vi "uTTA_Main_Temperature_Control.vi"() -> ()   [LabVIEW 2021]
uses:
  uTTA_Device_Driver/uTTA_Controls/CTL_uTTA_MeasurementStates.ctl
  <vilib>/Utility/miscctls.llb/LVPointTypeDef.ctl
  uTTA_Device_Driver/uTTA_Controls/CTL_uTTA_OperatingMode.ctl
  uTTA_Device_Driver/uTTA_Controls/CTL_uTTA_AnalogParameter.ctl
  <vilib>/Utility/error.llb/DialogType.ctl
  uTTA_Device_Driver/uTTA_SubVi/Serial_Port/uTTA_GV_Serial_Monitor.vi
panel:
  out "Updated":dbl
  out "Stable Time":dbl
  in  "Set Point":dbl
  out "Temperature":dbl
  in  "Update_Time":dbl=0.5
  out "uTTA_CalData":T1(array[cluster])
  out "ADC Overrange":bool[](array[boolean])
  out "GUI State":string="EXIT"
  out "Heating Power":dbl format="%#_3pW"
  out "Total Runtime":timestamp=timestamp(-3599.4283056259155 s since 1904-01-01) format="%<%H:%M:%S>T"
  out "Measurement Started":timestamp=timestamp(3793474800.1504135 s since 1904-01-01) format="%<%X>T"
  out "Diode Voltages":T2(graph)
  out "Temp":T3(graph)
  out "Measurement State":T4=enum."Cooling" caption="uTTA State"
  in  "Tab Control":T5(tab)
  out "ADC1L_Range":dbl caption="Lower Limit" format="%.2pV"
  out "ADC1H_Range":dbl caption="Upper Limit" format="%.2pV"
  in  "CH1-2 Offset":dbl(slide)=-0.4 scale=-2.5..2.5 scale format="%.2pV"
  out "ADC0H_Range":dbl caption="Upper Limit" format="%.2pV"
  out "ADC0L_Range":dbl caption="Lower Limit" format="%.2pV"
  in  "CH0 Offset":dbl(slide)=-0.63 scale=-2.5..2.5 scale format="%.2pV"
  in  "Sense Current":dbl(slide)=0.01 caption="CH0" min=0.0 max=0.011 step=0.0001 scale=0.0..0.011 scale format="%.1pA"
  in  "µTTA Port":refnum<visa-resource-name>="COM3"
  in  "Connect":bool
  in  "Disconnect":bool
  in  "Heating":u16(ring) items=["PGA = 0", "PGA = 1", "PGA = 2", "PGA = 3"]
  in  "Start":bool
  in  "Stop":bool
  in  "Autoscroll":bool
  out "Serial Monitor OUT":string
  in  "Serial Monitor":bool
  out "RunTime Error":errorcluster
  out "Exit Error":errorcluster
  out "Device Info":string
  # "Measurement\nRange"
  # "Measurement \nRange"
  # "Channel Offset"
  # "Sense Current"
  # "PGA"
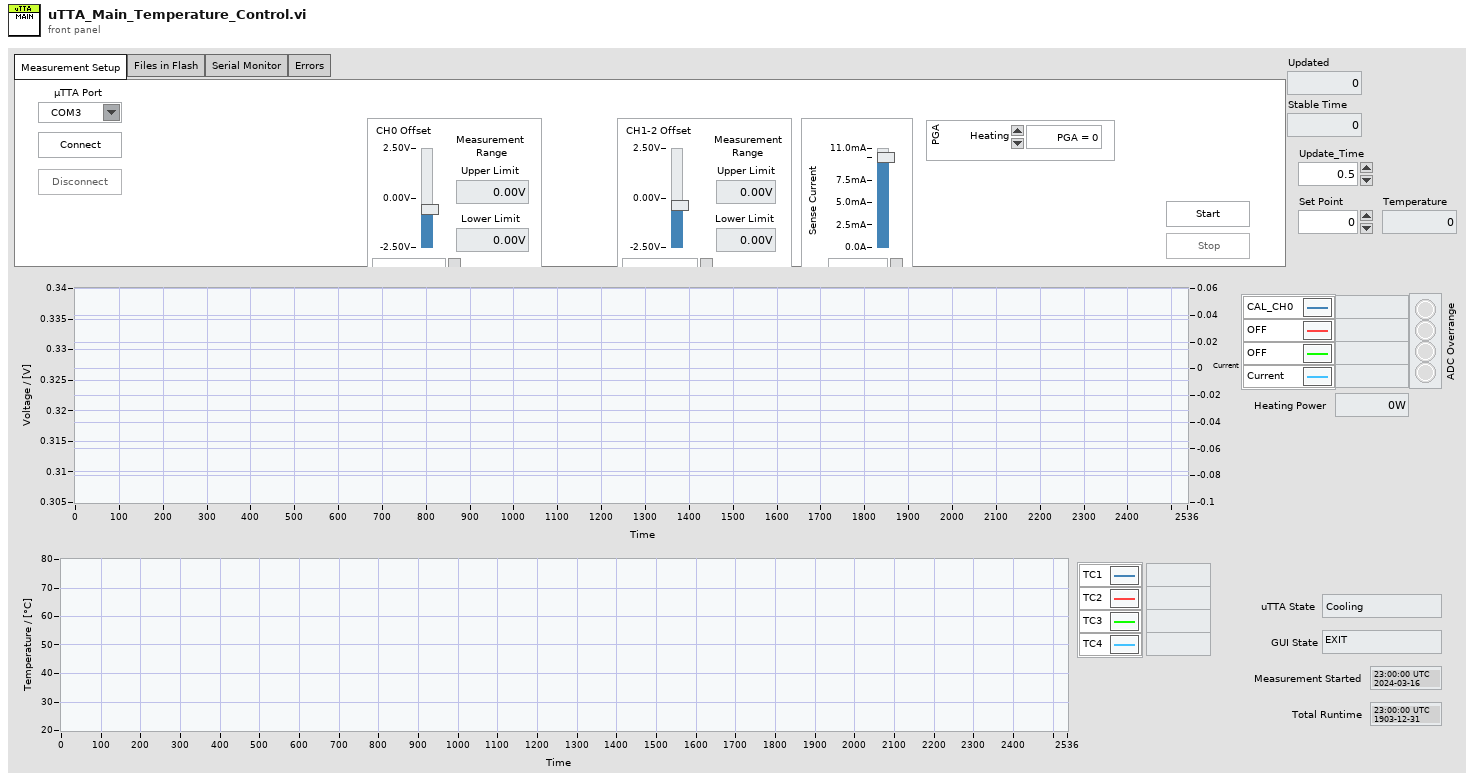
[diagram p1: front panel]
types:
  T1 = cluster{"Diff Gain":dbl, "Offset":dbl[], "Gain":dbl[]}[]
  T2 = cluster{"Diode Voltage":dbl, "Diode Voltage":dbl, "Diode Voltage":dbl, "Current":dbl}
  T3 = cluster{"Diode Voltage":dbl, "Diode Voltage":dbl, "Diode Voltage":dbl, "Diode Voltage":dbl}
  T4 = typedef "CTL_uTTA_MeasurementStates.ctl" = enum16{"Idle", "Init", "GPPowerCheck", "InitMeasFile", "Preheating", "PrepHeating", "Heating", "PrepCooling", "Cooling", "Deinit", "CloseLog", "Cal_Init", "Cal_GDPowerOn", "Cal_GDPowerCheck", "Cal_Cal", "Cal_Deinit"}
  T5 = enum32{"Measurement Setup", "Files in Flash", "Serial Monitor", "Errors"}
  T6 = typedef "LVPointTypeDef.ctl" = cluster{"Horizontal":i16, "Vertical":i16}
  T7 = typedef "CTL_uTTA_AnalogParameter.ctl" = enum16{"ISEN", "SPARE", "VOFF"}
  T8 = enum8{"Enabled", "Disabled", "Disabled and Grayed Out"}
  T9 = typedef "CTL_uTTA_OperatingMode.ctl" = enum16{"NORMAL", "TEST_MODE", "TEMP_CONTROL"}
  T10 = cluster{"Diode Voltage":dbl, "Diode Voltage":dbl, "Diode Voltage":dbl, "Current":dbl}[]
  T11 = cluster{"Diode Voltage":dbl, "Diode Voltage":dbl, "Diode Voltage":dbl, "Diode Voltage":dbl}[]
  T12 = cluster{"Measurement State":T4, "Diode Voltages":dbl[], "Current":dbl, "Temperatures":dbl[], "NewData":bool, "ADC Overrange":bool[]}
  T13 = typedef "DialogType.ctl" = u16
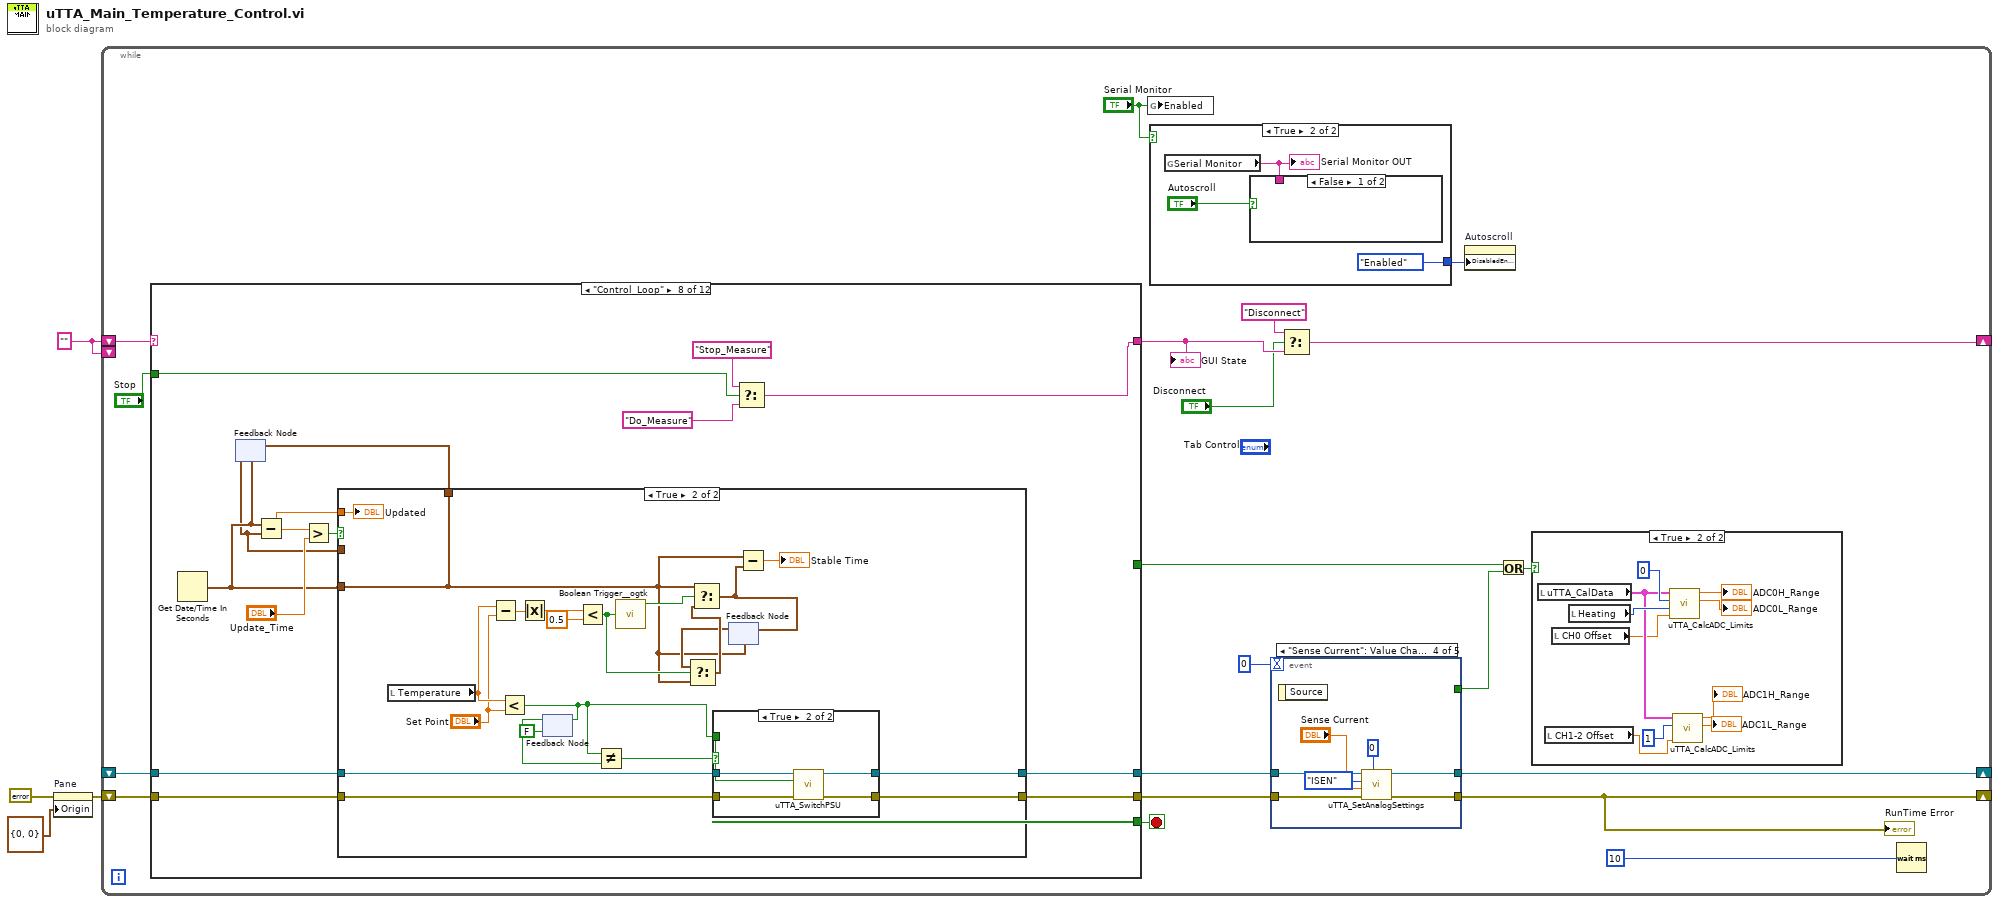
[diagram p0: block diagram]
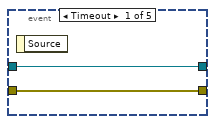
[diagram p3: hidden frame]
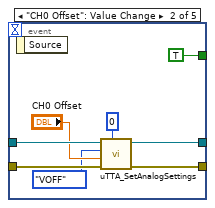
[diagram p4: hidden frame]
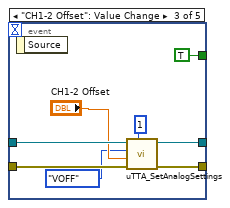
[diagram p5: hidden frame]
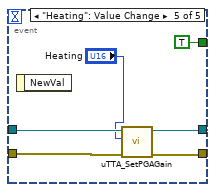
[diagram p6: hidden frame]
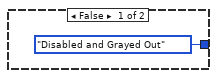
[diagram p7: hidden frame]
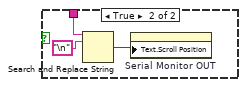
[diagram p8: hidden frame]
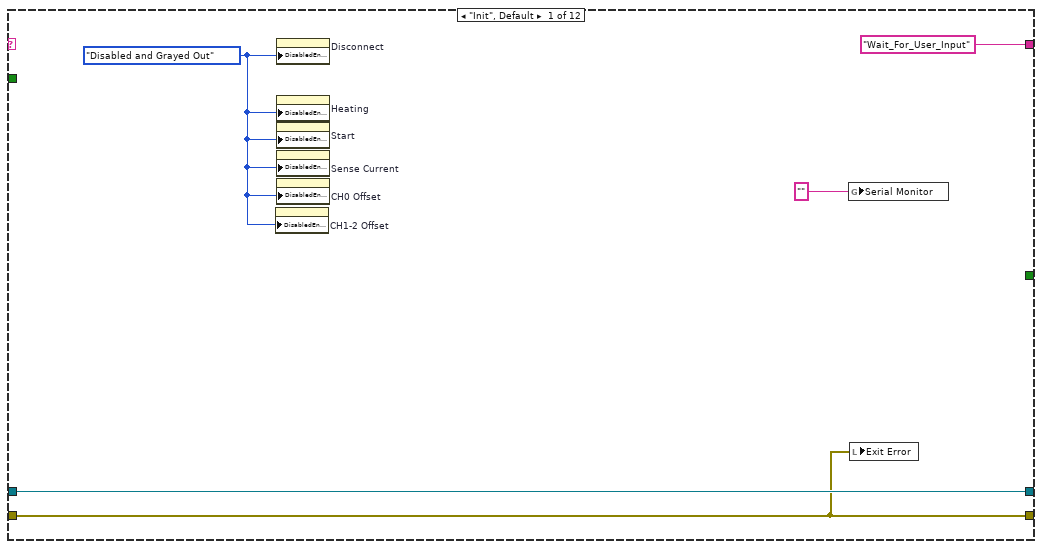
[diagram p9: hidden frame]
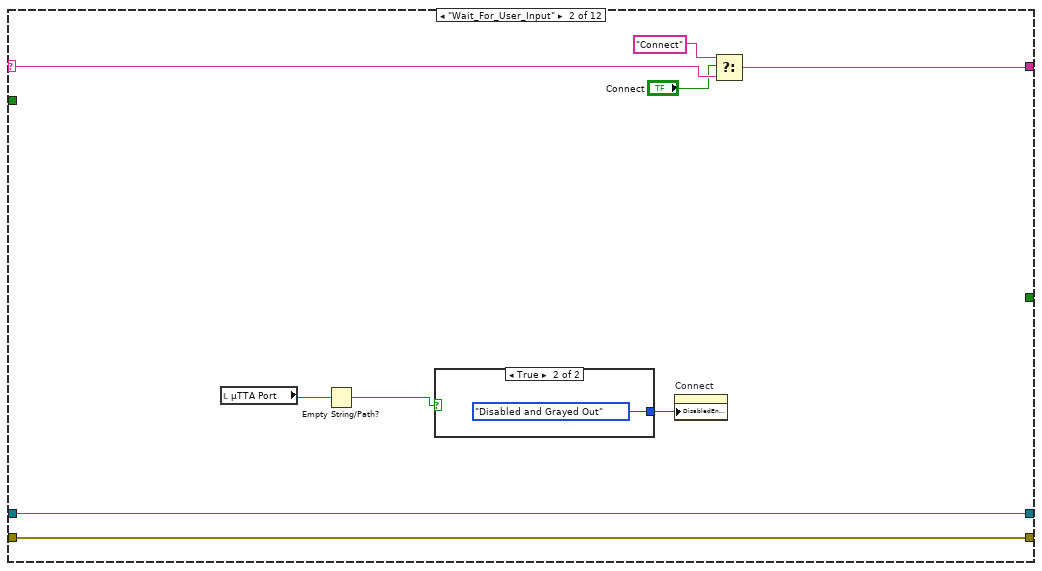
[diagram p10: hidden frame]
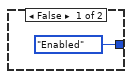
[diagram p11: hidden frame]
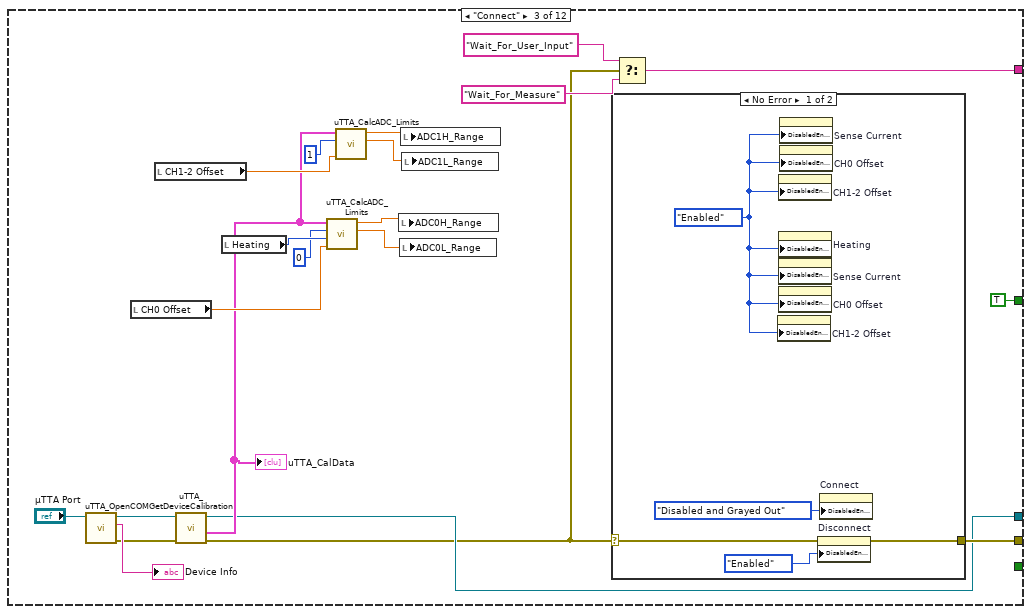
[diagram p12: hidden frame]
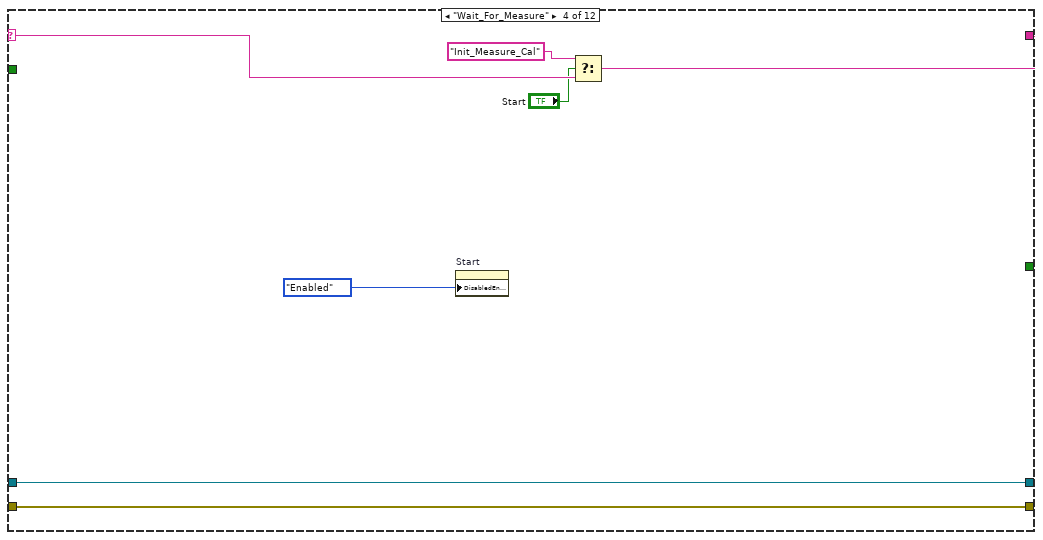
[diagram p14: hidden frame]
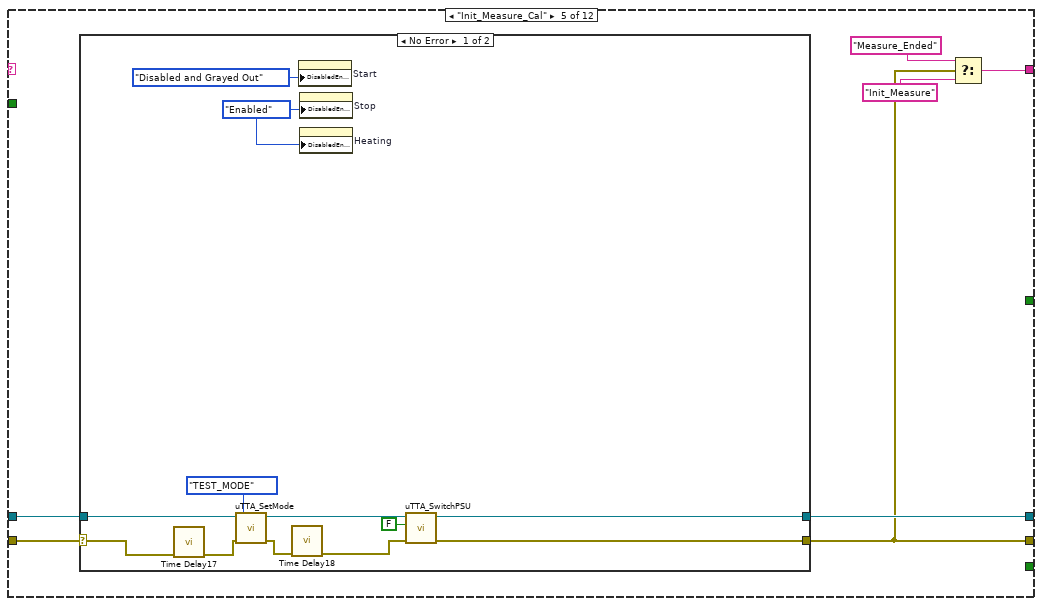
[diagram p15: hidden frame]
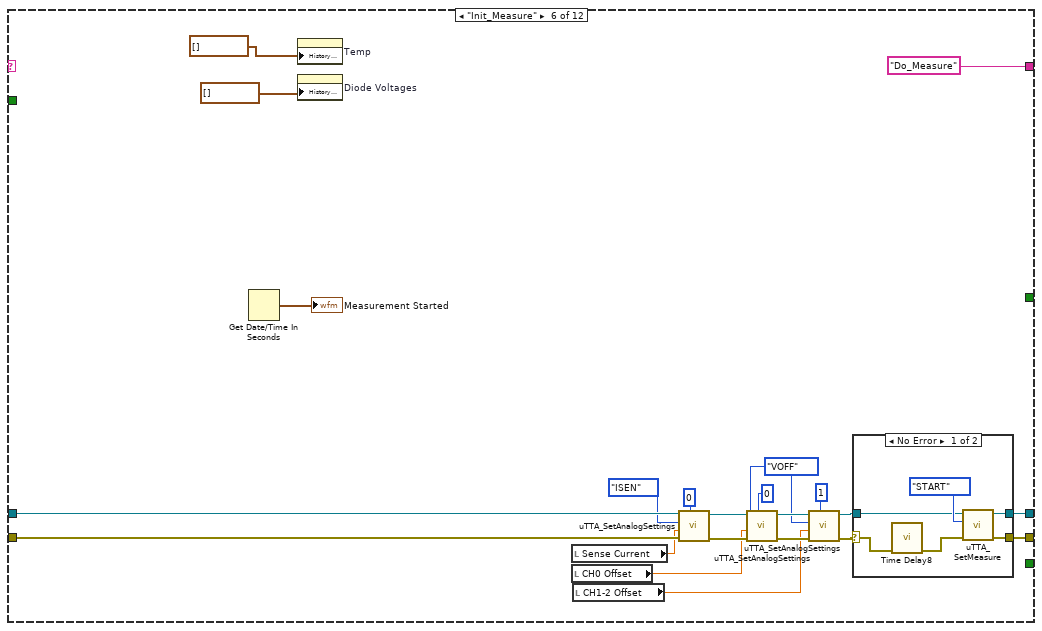
[diagram p17: hidden frame]
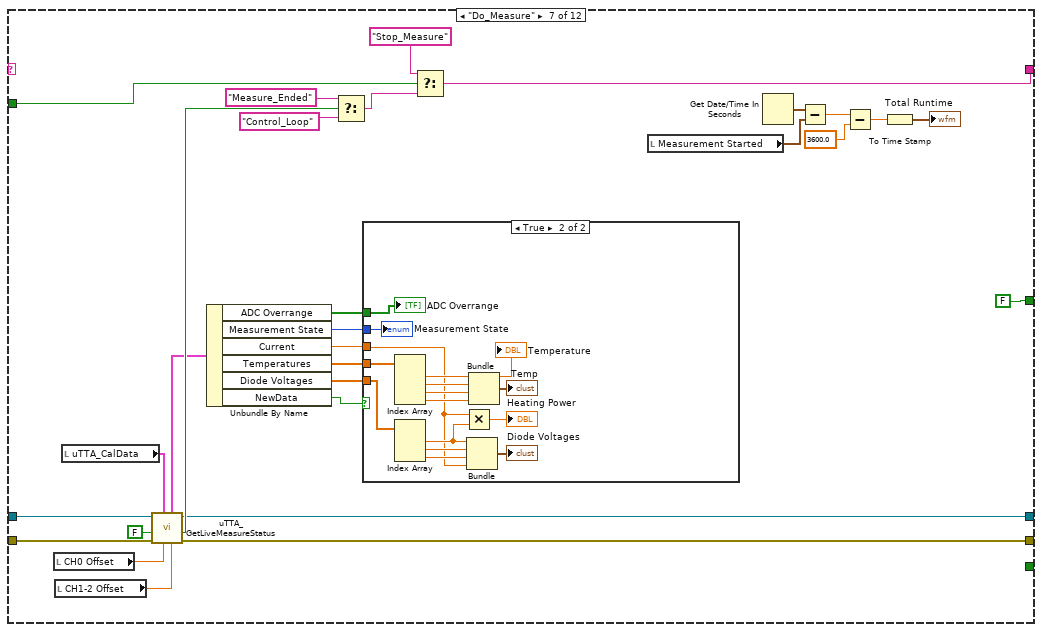
[diagram p19: hidden frame]
diagram:
  w1 = "" ("Identity")
  n1 = property on="Pane" class="Pane"(error in=errorcluster {"status"=FALSE, "code"=0, "source"=""} ("error out"), "Origin"=T6 {"Horizontal"=0, "Vertical"=0}) -> (error out=w2:errorcluster)  [unwired: 1 in, 1 out]
  n2 = while {
    shift-right: [w18] -> _
    shift-left: w1 -> [w24]
    shift-right: [w10] -> _
    shift-left: _ -> [w23]
    shift-right: [w8] -> _
    shift-left: w2 -> [w22]
    shift-left: w1 -> [_]
    stop <- w21 stop-if-true
    n3 = case shown="\"Control_Loop\"" w24 {
      selector: w24 -> [_ w85 _ w121 _ _ _ _ _ _ _ w287]
      tunnel: ["Wait_For_User_Input" w86 w104 w120 w124 "Do_Measure" ("t") w190 w223 "Measure_Ended" ("t") "Wait_For_Measure" ("t") "EXIT" w287] -> w19
      tunnel: [w76 w83 w90 w118 w129 w165 w181 w228 w265 w272 refnum<visa-resource-name> refnum ("VISA out") w286] -> w11
      tunnel: w23 -> [w76 w83 _ w118 w128 w160 w202 w229 w267 w272 w281 w286]
      tunnel: w22 -> [w75 w82 _ w116 w127 w161 w201 w226 w266 w271 w282 w285]
      tunnel: [w75 w82 w107 w116 w123 w164 w180 w227 w264 w271 w278 w285] -> w9
      tunnel: [_ _ _ _ _ _ _ _ _ _ _ TRUE] -> w21
      tunnel: "Stop" -> [_ _ _ _ _ _ w193 w224 _ _ _ _]
      tunnel: [_ _ TRUE _ _ _ FALSE _ _ _ _ _] -> w5
      frame "Init", Default {
        w73 = T8."Disabled and Grayed Out" ("Disabled")
        n4 = property on="CH1-2 Offset" class="Slide (strict)"("DisabledEnum"=w73) -> ()  [unwired: 2 in, 2 out]
        n5 = property on="Disconnect" class="Bool"("DisabledEnum"=w73) -> ()  [unwired: 2 in, 2 out]
        n6 = property on="Heating" class="Ring (strict)"("DisabledEnum"=w73) -> ()  [unwired: 2 in, 2 out]
        n7 = property on="Start" class="Bool"("DisabledEnum"=w73) -> ()  [unwired: 2 in, 2 out]
        n8 = property on="Sense Current" class="Slide (strict)"("DisabledEnum"=w73) -> ()  [unwired: 2 in, 2 out]
        n9 = property on="CH0 Offset" class="Slide (strict)"("DisabledEnum"=w73) -> ()  [unwired: 2 in, 2 out]
        n10 = global write "uTTA_GV_Serial_Monitor.vi" "Serial Monitor"("" ("Received")) -> ()
        n11 = local write "Exit Error"(w75) -> ()
      }
      frame "Wait_For_User_Input" {
        n12 = local read "µTTA Port"() -> (w81:refnum<visa-resource-name>)
        n13 = Empty String/Path?(string/path=w81) -> (empty?=w78:bool)
        n14 = case shown="True" w78 {
          tunnel: [T8."Enabled" ("Disabled") T8."Disabled and Grayed Out" ("Disabled")] -> w79
          frame False {
          }
          frame True {
          }
        }
        n15 = property on="Connect" class="Bool"("DisabledEnum"=w79) -> ()  [unwired: 2 in, 2 out]
        n16 = Select(t="Connect", s="Connect", f=w85) -> (s? t:f=w86:string)
      }
      frame "Connect" {
        n17 = call "uTTA_OpenCOM.vi"("VISA in"="µTTA Port") -> ("error out"=w93:errorcluster, "Identity"=→"Device Info":string, "VISA out"=w94:refnum<visa-resource-name>)  [unwired: 8 in]
        n18 = local read "CH0 Offset"() -> (w96:dbl)
        n19 = local read "CH1-2 Offset"() -> (w101:dbl)
        n20 = call "uTTA_GetDeviceCalibration.vi"("error in"=w93, "VISA Refnum in"=w94) -> ("error out"=w89:errorcluster, "uTTA_CalData"=w92:T1, "VISA Refnum out"=w90:refnum<visa-resource-name>)  [unwired: 2 in, 1 out]
        "uTTA_CalData" <- w92
        n21 = local read "Heating"() -> (w103:u16)
        n22 = call "uTTA_CalcADC_Limits.vi"("Offset Voltage"=w96, "PGA_Setting"=w103, "Channel Number"=u32 0, "uTTA_CalData"=w92) -> ("Range Low End"=w97:dbl, "Range High End"=w98:dbl)  [unwired: 6 in]
        n23 = call "uTTA_CalcADC_Limits.vi"("Offset Voltage"=w101, "Channel Number"=u32 1, "uTTA_CalData"=w92) -> ("Range Low End"=w99:dbl, "Range High End"=w100:dbl)  [unwired: 7 in]
        n24 = local write "ADC0H_Range"(w98) -> ()
        n25 = local write "ADC0L_Range"(w97) -> ()
        n26 = local write "ADC1H_Range"(w100) -> ()
        n27 = local write "ADC1L_Range"(w99) -> ()
        n28 = case shown="No Error" w89 {
          selector: w89 -> [w112 w115]
          tunnel: [w113 w115] -> w107
          frame No Error {
            w110 = T8."Enabled" ("Disabled")
            n29 = property on="CH1-2 Offset" class="Slide (strict)"("DisabledEnum"=w110) -> ()  [unwired: 2 in, 2 out]
            n30 = property on="CH1-2 Offset" class="Slide (strict)"("DisabledEnum"=w110) -> ()  [unwired: 2 in, 2 out]
            n31 = property on="Heating" class="Ring (strict)"("DisabledEnum"=w110) -> ()  [unwired: 2 in, 2 out]
            n32 = property on="Sense Current" class="Slide (strict)"("DisabledEnum"=w110) -> ()  [unwired: 2 in, 2 out]
            n33 = property on="CH0 Offset" class="Slide (strict)"("DisabledEnum"=w110) -> ()  [unwired: 2 in, 2 out]
            n34 = property on="Sense Current" class="Slide (strict)"("DisabledEnum"=w110) -> ()  [unwired: 2 in, 2 out]
            n35 = property on="CH0 Offset" class="Slide (strict)"("DisabledEnum"=w110) -> ()  [unwired: 2 in, 2 out]
            n36 = property on="Disconnect" class="Bool"(error in=w112, "DisabledEnum"=T8."Enabled" ("Disabled")) -> (error out=w113:errorcluster)  [unwired: 1 in, 1 out]
            n37 = property on="Connect" class="Bool"("DisabledEnum"=T8."Disabled and Grayed Out" ("Disabled")) -> ()  [unwired: 2 in, 2 out]
          }
          frame Error {
          }
        }
        n38 = Select(t="Wait_For_User_Input", s=w89, f="Wait_For_Measure" ("t")) -> (s? t:f=w104:string)
      }
      frame "Wait_For_Measure" {
        n39 = property on="Start" class="Bool"("DisabledEnum"=T8."Enabled" ("Disabled")) -> ()  [unwired: 2 in, 2 out]
        n40 = Select(t="Init_Measure_Cal", s="Start", f=w121) -> (s? t:f=w120:string)
      }
      frame "Init_Measure_Cal" {
        n41 = case shown="No Error" w127 {
          selector: w127 -> [w138 w142]
          tunnel: w128 -> [w137 w143]
          tunnel: [w132 w143] -> w129
          tunnel: [w131 w142] -> w123
          frame No Error {
            w136 = T8."Enabled" ("Disabled")
            n42 = call "Time Delay17"("error in (no error)"=w138) -> ("error out"=w139:errorcluster)  [unwired: 10 in]
            n43 = call "uTTA_SetMode.vi"("error in"=w139, "OperatingMode"=CTL_uTTA_OperatingMode."TEST_MODE", "VISA Refnum in"=w137) -> ("error out"=w140:errorcluster, "VISA Refnum out"=w134:refnum<visa-resource-name>)  [unwired: 2 in, 1 out]
            n44 = call "Time Delay18"("error in (no error)"=w140) -> ("error out"=w133:errorcluster)  [unwired: 10 in]
            n45 = property on="Start" class="Bool"("DisabledEnum"=T8."Disabled and Grayed Out" ("Disabled")) -> ()  [unwired: 2 in, 2 out]
            n46 = property on="Stop" class="Bool"("DisabledEnum"=w136) -> ()  [unwired: 2 in, 2 out]
            n47 = property on="Heating" class="Ring (strict)"("DisabledEnum"=w136) -> ()  [unwired: 2 in, 2 out]
            n48 = call "uTTA_SwitchPSU.vi"("error in"=w133, "PSU Enable"=FALSE, "VISA Refnum in"=w134) -> ("error out"=w131:errorcluster, "VISA Refnum out"=w132:refnum<visa-resource-name>)  [unwired: 2 in, 1 out]
          }
          frame Error {
          }
        }
        n49 = Select(t="Measure_Ended", s=w123, f="Init_Measure" ("t")) -> (s? t:f=w124:string)
      }
      frame "Init_Measure" {
        w147 = CTL_uTTA_AnalogParameter."VOFF" ("Parameter")
        n50 = Get Date/Time In Seconds() -> (seconds since 1Jan1904=→"Measurement Started":timestamp)
        n51 = property on="Temp" class="WFChart (strict)"("History Data"=T11 []) -> ()  [unwired: 2 in, 2 out]
        n52 = property on="Diode Voltages" class="WFChart (strict)"("History Data"=T10 []) -> ()  [unwired: 2 in, 2 out]
        n53 = local read "Sense Current"() -> (w150:dbl)
        n54 = local read "CH0 Offset"() -> (w151:dbl)
        n55 = local read "CH1-2 Offset"() -> (w149:dbl)
        n56 = call "uTTA_SetAnalogSettings.vi"("Number"=u32 0, "error in"=w161, "Set Value"=w150, "Parameter"=CTL_uTTA_AnalogParameter."ISEN", "VISA Refnum in"=w160) -> ("error out"=w157:errorcluster, "VISA Refnum out"=w156:refnum<visa-resource-name>)  [unwired: 2 in, 1 out]
        n57 = call "uTTA_SetAnalogSettings.vi"("Number"=u32 0, "error in"=w157, "Set Value"=w151, "Parameter"=w147, "VISA Refnum in"=w156) -> ("error out"=w155:errorcluster, "VISA Refnum out"=w154:refnum<visa-resource-name>)  [unwired: 2 in, 1 out]
        n58 = call "uTTA_SetAnalogSettings.vi"("Number"=u32 1, "error in"=w155, "Set Value"=w149, "Parameter"=w147, "VISA Refnum in"=w154) -> ("error out"=w152:errorcluster, "VISA Refnum out"=w153:refnum<visa-resource-name>)  [unwired: 2 in, 1 out]
        n59 = case shown="No Error" w152 {
          selector: w152 -> [w167 w172]
          tunnel: w153 -> [w166 w173]
          tunnel: [w171 w173] -> w165
          tunnel: [w170 w172] -> w164
          frame No Error {
            n60 = call "Time Delay8"("error in (no error)"=w167) -> ("error out"=w168:errorcluster)  [unwired: 10 in]
            n61 = call "uTTA_SetMeasure.vi"("error in"=w168, "Action"=enum16{"STOP", "START"}."START", "VISA Refnum in"=w166) -> ("error out"=w170:errorcluster, "VISA Refnum out"=w171:refnum<visa-resource-name>)  [unwired: 2 in, 1 out]
          }
          frame Error {
          }
        }
      }
      frame "Do_Measure" {
        n62 = local read "CH0 Offset"() -> (w178:dbl)
        n63 = local read "CH1-2 Offset"() -> (w177:dbl)
        n64 = local read "uTTA_CalData"() -> (w179:T1)
        n65 = call "uTTA_GetLiveMeasureStatus.vi"("CH1&2 Offset Voltage"=w177, "CH0 Offset Voltage"=w178, "uTTA_CalData"=w179, "error in"=w201, "CalibrationMode"=FALSE, "VISA Refnum in"=w202) -> ("error out"=w180:errorcluster, "Measurement Completed"=w200:bool, "VISA Refnum out"=w181:refnum<visa-resource-name>, "Measurement Data"=w198:T12)  [unwired: 1 in, 1 out]
        n66 = Unbundle By Name(w198) -> ("ADC Overrange"=w182:bool[], "Measurement State"=w197:T4, "Current"=w196:dbl, "Temperatures"=w195:dbl[], "Diode Voltages"=w194:dbl[], "NewData"=w189:bool)
        n67 = Select(t="Measure_Ended", s=w200, f="Control_Loop") -> (s? t:f=w192:string)
        n68 = case shown="True" w189 {
          tunnel: w197 -> [_ w217]
          tunnel: w196 -> [_ w205]
          tunnel: w195 -> [_ w203]
          tunnel: w194 -> [_ w209]
          tunnel: w182 -> [_ w204]
          frame False {
          }
          frame True {
            n69 = Index Array(array=w203) -> (element #1=w215:dbl, element #2=w214:dbl, element #3=w213:dbl, element #4=w212:dbl)  [unwired: 4 in]
            "Temperature" <- w215
            n70 = Index Array(array=w209) -> (element #1=w208:dbl, element #2=w207:dbl, element #3=w206:dbl)  [unwired: 3 in]
            n71 = Multiply(x=w205, y=w208) -> (x*y=→"Heating Power":dbl)
            n72 = Bundle("Diode Voltage"=w208, "Diode Voltage"=w207, "Diode Voltage"=w206, "Current"=w205) -> (→"Diode Voltages":T2)  [unwired: 1 in]
            n73 = Bundle("Diode Voltage"=w215, "Diode Voltage"=w214, "Diode Voltage"=w213, "Diode Voltage"=w212) -> (→"Temp":T3)  [unwired: 1 in]
            "Measurement State" <- w217
            "ADC Overrange" <- w204
          }
        }
        n74 = Select(t="Stop_Measure", s=w193, f=w192) -> (s? t:f=w190:string)
        n75 = local read "Measurement Started"() -> (w188:timestamp)
        n76 = Get Date/Time In Seconds() -> (seconds since 1Jan1904=w183:timestamp)
        n77 = Subtract(x=w183, y=w188) -> (x-y=w185:dbl)
        n78 = Subtract(x=w185, y=3600.0) -> (x-y=w186:dbl)
        n79 = To Time Stamp(1:w186) -> (0:→"Total Runtime":timestamp)
      }
      frame "Control_Loop" {
        n80 = Get Date/Time In Seconds() -> (seconds since 1Jan1904=w221:timestamp)
        n81 = feedback #1(w221) -> (w218:timestamp)
        n82 = Subtract(x=w221, y=w218) -> (x-y=w220:dbl)
        n83 = Greater?(x=w220, y="Update_Time") -> (0:w230:bool)
        n84 = case shown="True" w230 {
          tunnel: w229 -> [w234 w255]
          tunnel: [w234 w253] -> w228
          tunnel: [w233 w252] -> w227
          tunnel: w226 -> [w233 w254]
          tunnel: w221 -> [_ w235]
          tunnel: w220 -> [_ w236]
          tunnel: [w232 w235] -> w219
          tunnel: w218 -> [w232 _]
          frame False {
          }
          frame True {
            n85 = local read "Temperature"() -> (w251:dbl)
            n86 = Subtract(x=w251, y="Set Point") -> (x-y=w249:dbl)
            n87 = Less?(x=w251, y="Set Point") -> (x < y?=w238:bool)
            n88 = Absolute Value(x=w249) -> (abs(x)=w248:dbl)
            n89 = feedback #2(FALSE) -> (w239:bool)
            n90 = feedback-in #2(w238) -> ()
            n91 = Less?(x=w248, y=0.5) -> (x < y?=w242:bool)
            n92 = Not Equal?(x=w238, y=w239) -> (x != y?=w237:bool)
            n93 = call <userlib>:"Boolean Trigger__ogtk.vi"("Boolean Input"=w242) -> ("Rising Edge"=w246:bool)  [unwired: 1 in, 1 out]
            n94 = case shown="True" w237 {
              tunnel: w255 -> [w257 w262]
              tunnel: w254 -> [w256 w261]
              tunnel: [w257 w260] -> w253
              tunnel: [w256 w259] -> w252
              tunnel: w238 -> [_ w258]
              frame False {
              }
              frame True {
                n95 = call "uTTA_SwitchPSU.vi"("error in"=w261, "PSU Enable"=w258, "VISA Refnum in"=w262) -> ("error out"=w259:errorcluster, "VISA Refnum out"=w260:refnum<visa-resource-name>)  [unwired: 2 in, 1 out]
              }
            }
            n96 = feedback #3(w235) -> (w241:timestamp)
            n97 = Select(t=w241, s=w242, f=w235) -> (s? t:f=w243:timestamp)
            n98 = Select(t=w235, s=w246, f=w243) -> (s? t:f=w245:timestamp)
            n99 = feedback-in #3(w245) -> ()
            n100 = Subtract(x=w235, y=w245) -> (x-y=→"Stable Time":dbl)
            "Updated" <- w236
          }
        }
        n101 = feedback-in #1(w219) -> ()
        n102 = Select(t="Stop_Measure", s=w224, f="Do_Measure" ("t")) -> (s? t:f=w223:string)
      }
      frame "Stop_Measure" {
        n103 = call "uTTA_SetMeasure.vi"("error in"=w266, "Action"=enum16{"STOP", "START"}."STOP", "VISA Refnum in"=w267) -> ("error out"=w264:errorcluster, "VISA Refnum out"=w265:refnum<visa-resource-name>)  [unwired: 2 in, 1 out]
      }
      frame "Measure_Ended" {
        n104 = property on="Heating" class="Ring (strict)"("DisabledEnum"=T8."Enabled" ("Disabled")) -> ()  [unwired: 2 in, 2 out]
        n105 = property on="Start" class="Bool"("DisabledEnum"=T8."Enabled" ("Disabled")) -> ()  [unwired: 2 in, 2 out]
        n106 = property on="Stop" class="Bool"("DisabledEnum"=T8."Disabled and Grayed Out" ("Disabled")) -> ()  [unwired: 2 in, 2 out]
      }
      frame "Disconnect" {
        w277 = T13 0 items=["no dialog", "OK message", "continue or stop message", "OK message + warnings", "continue/stop + warnings"] ("type of dialog (OK msg:1)")
        n107 = VISA Close(VISA resource name=w281, error in (no error)=w282) -> (error out=w275:errorcluster)
        "Exit Error" <- w275
        n108 = property on="Connect" class="Bool"("DisabledEnum"=T8."Enabled" ("Disabled")) -> ()  [unwired: 2 in, 2 out]
        n109 = property on="Disconnect" class="Bool"("DisabledEnum"=T8."Disabled and Grayed Out" ("Disabled")) -> ()  [unwired: 2 in, 2 out]
        n110 = call <vilib>:"Simple Error Handler.vi"("type of dialog (OK msg:1)"=w277, "error in (no error)"=w275) -> ("error out"=w278:errorcluster)  [unwired: 3 in, 4 out]
      }
      frame "EXIT" {
      }
    }
    "GUI State" <- w19
    n111 = global write "uTTA_GV_Serial_Monitor.vi" "Enabled"("Serial Monitor") -> ()
    n112 = case shown="True" "Serial Monitor" {
      tunnel: [T8."Disabled and Grayed Out" ("Disabled") T8."Enabled" ("Disabled")] -> w14
      frame False {
      }
      frame True {
        n113 = global read "uTTA_GV_Serial_Monitor.vi" "Serial Monitor"() -> (w69:string)
        "Serial Monitor OUT" <- w69
        n114 = case shown="False" "Autoscroll" {
          tunnel: w69 -> [_ w72]
          frame False {
          }
          frame True {
            n115 = Search and Replace String(input string=w72, search string="\n") -> (number of replacements=w70:i32)  [unwired: 6 in, 3 out]
            n116 = property on="Serial Monitor OUT" class="Str"("Text.Scroll Position"=w70) -> ()  [unwired: 2 in, 2 out]
          }
        }
      }
    }
    n117 = event shown="[3] \"Sense Current\": Value Change" {
      selector: _ -> [_ _ _ _ _]
      dyn-events: _ -> [_ _ _ _ _]
      timeout: 0 -> [_ _ _ _ _]
      tunnel: w11 -> [w36 w44 w52 w59 w65]
      tunnel: w9 -> [w35 w43 w51 w58 w63]
      tunnel: [w36 w42 w50 w57 w64] -> w10
      tunnel: [w35 w41 w49 w56 w62] -> w8
      tunnel: [_ TRUE TRUE _ TRUE] -> w6
      event Timeout {
        n118 = event-data() -> ()  [unwired: 1 in, 1 out]
      }
      event "CH0 Offset": Value Change {
        n119 = event-data() -> ()  [unwired: 1 in, 1 out]
        n120 = call "uTTA_SetAnalogSettings.vi"("Number"=u32 0, "error in"=w43, "Set Value"="CH0 Offset", "Parameter"=CTL_uTTA_AnalogParameter."VOFF", "VISA Refnum in"=w44) -> ("error out"=w41:errorcluster, "VISA Refnum out"=w42:refnum<visa-resource-name>)  [unwired: 2 in, 1 out]
      }
      event "CH1-2 Offset": Value Change {
        n121 = event-data() -> ()  [unwired: 1 in, 1 out]
        n122 = call "uTTA_SetAnalogSettings.vi"("Number"=u32 1, "error in"=w51, "Set Value"="CH1-2 Offset", "Parameter"=CTL_uTTA_AnalogParameter."VOFF", "VISA Refnum in"=w52) -> ("error out"=w49:errorcluster, "VISA Refnum out"=w50:refnum<visa-resource-name>)  [unwired: 2 in, 1 out]
      }
      event "Sense Current": Value Change {
        n123 = event-data() -> ()  [unwired: 1 in, 1 out]
        n124 = call "uTTA_SetAnalogSettings.vi"("Number"=u32 0, "error in"=w58, "Set Value"="Sense Current", "Parameter"=CTL_uTTA_AnalogParameter."ISEN", "VISA Refnum in"=w59) -> ("error out"=w56:errorcluster, "VISA Refnum out"=w57:refnum<visa-resource-name>)  [unwired: 2 in, 1 out]
      }
      event "Heating": Value Change {
        n125 = event-data() -> ()  [unwired: 1 in, 1 out]
        n126 = call "uTTA_SetPGAGain.vi"("error in"=w63, "PGA Gain"="Heating", "VISA Refnum in"=w65) -> ("error out"=w62:errorcluster, "VISA Refnum out"=w64:refnum<visa-resource-name>)  [unwired: 5 in, 2 out]
      }
    }
    "RunTime Error" <- w8
    n127 = Select(t="Disconnect", s="Disconnect", f=w19) -> (s? t:f=w18:string)
    n128 = property on="Autoscroll" class="Bool (strict)"("DisabledEnum"=w14) -> ()  [unwired: 2 in, 2 out]
    n129 = Or(x=w5, y=w6) -> (x .or. y?=w7:bool)
    n130 = case shown="True" w7 {
      frame False {
      }
      frame True {
        n131 = local read "uTTA_CalData"() -> (w27:T1)
        n132 = local read "CH1-2 Offset"() -> (w26:dbl)
        n133 = local read "CH0 Offset"() -> (w25:dbl)
        n134 = local read "Heating"() -> (w29:u16)
        n135 = call "uTTA_CalcADC_Limits.vi"("Offset Voltage"=w25, "PGA_Setting"=w29, "Channel Number"=u32 0, "uTTA_CalData"=w27) -> ("Range Low End"=→"ADC0L_Range":dbl, "Range High End"=→"ADC0H_Range":dbl)  [unwired: 6 in]
        n136 = call "uTTA_CalcADC_Limits.vi"("Offset Voltage"=w26, "Channel Number"=u32 1, "uTTA_CalData"=w27) -> ("Range Low End"=→"ADC1L_Range":dbl, "Range High End"=→"ADC1H_Range":dbl)  [unwired: 7 in]
      }
    }
    n137 = Wait (ms)(milliseconds to wait=u32 10) -> ()  [unwired: 1 out]
  }
